vi "cic_test_reconfigure.vi"() -> ()   [LabVIEW 2013]
panel:
  out "Waveform Graph out 2":i16[](graph)
  out "Waveform Graph out":dbl[](graph)
  out "Waveform Graph":dbl[](graph)
  out "# of Iterations":i32
  out "# of samples":i32
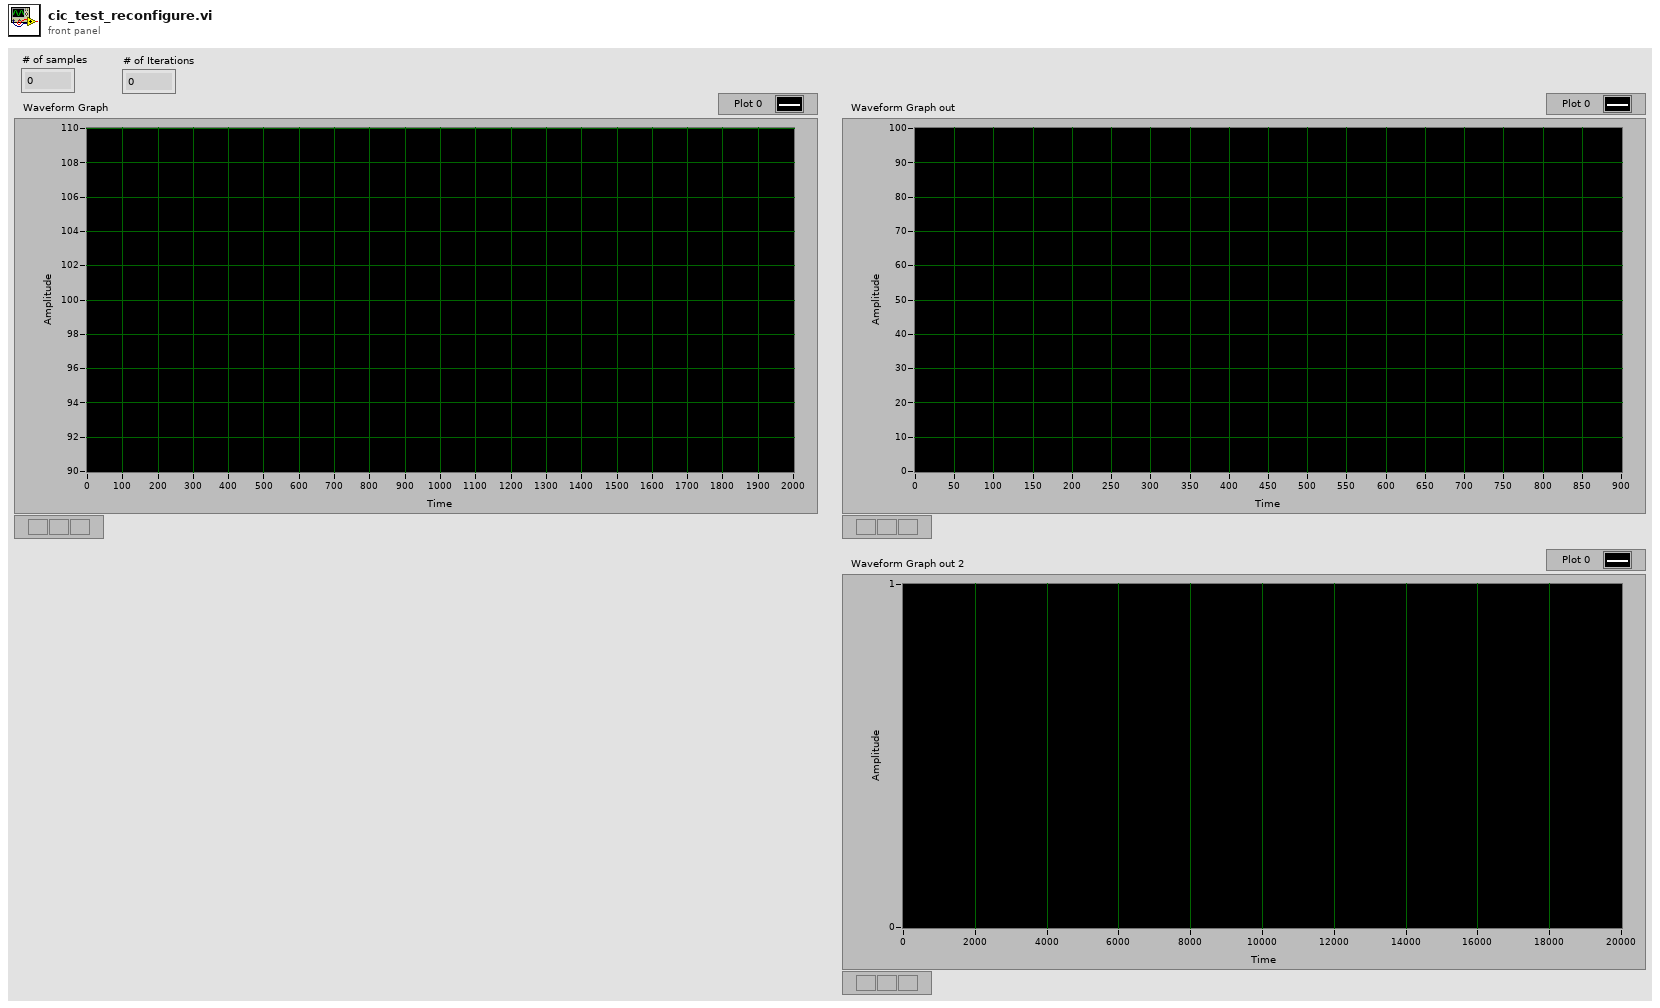
[diagram p1: front panel]
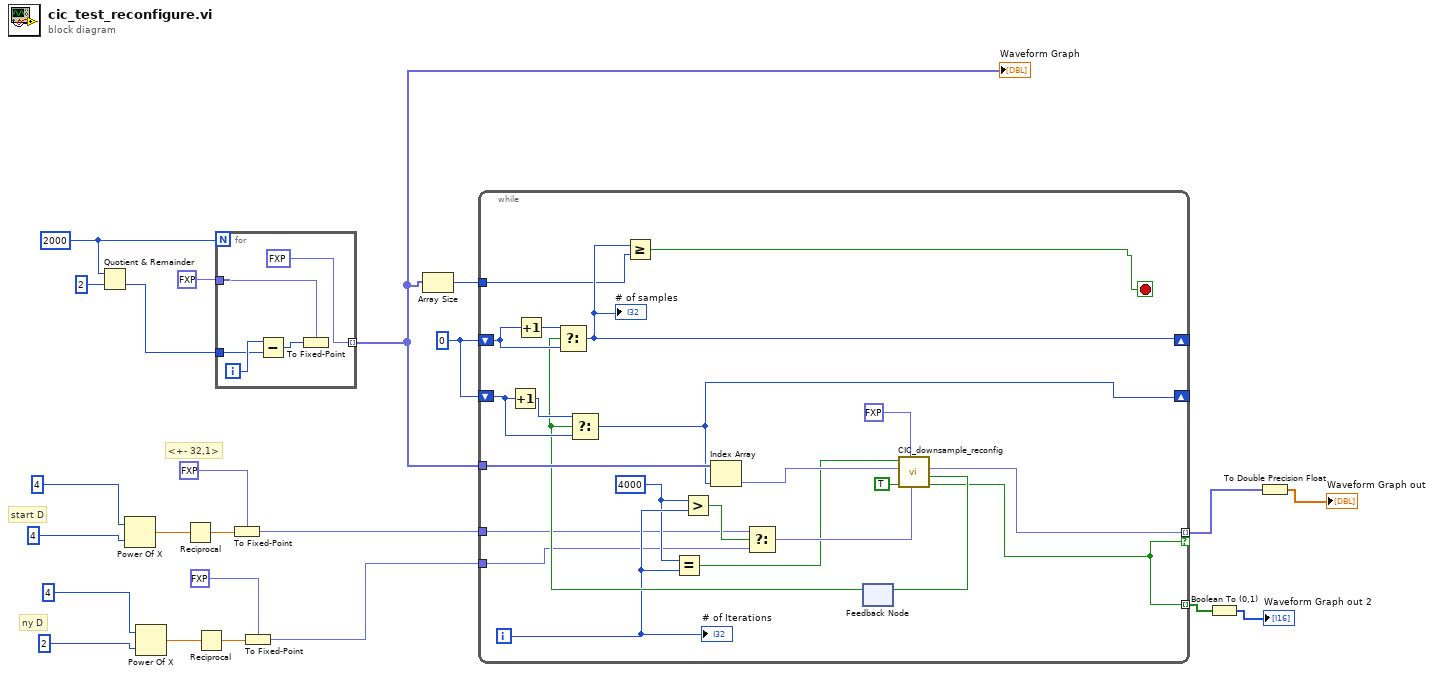
[diagram p0: block diagram]
diagram:
  w17 = 2000
  w21 = 0 ("samples")
  # "<+- 32,1>"
  # "ny D"
  # "start D"
  n1 = Quotient & Remainder(x=w17, y=2) -> (floor(x/y)=w15:i32)  [unwired: 1 out]
  n2 = Power Of X(1:4, 2:4) -> (0:w10:dbl)
  n3 = Power Of X(1:2, 2:4) -> (0:w4:dbl)
  n4 = Reciprocal(x=w10) -> (1/x=w9:dbl)
  n5 = Reciprocal(x=w4) -> (1/x=w5:dbl)
  n6 = for {
    N: w17 -> [_]
    tunnel: fxp<+/-,16,14> 0.0 ("fixed-point type") -> [w28]
    tunnel: [fxp<+/-,16,14> 100.0 ("fixed-point")] -> w18 mode=indexing
    tunnel: w15 -> [w26]
    i -> [w27]
    n7 = Subtract(x=w27, y=w26) -> (x-y=w25:i32)
    n8 = To Fixed-Point(fixed-point type=w28, number=w25) -> ()  [unwired: 1 out]
  }
  "Waveform Graph" <- w18
  n9 = To Fixed-Point(fixed-point type=fxp<+/-,32,1> 0.0 ("Gain"), number=w9) -> (fixed-point=w7:fxp<+/-,32,1>)
  n10 = To Fixed-Point(fixed-point type=fxp<+/-,32,1> 0.0 ("Gain"), number=w5) -> (fixed-point=w1:fxp<+/-,32,1>)
  n11 = Array Size(array=w18) -> (size(s)=w22:i32)
  n12 = while {
    tunnel: w18 -> [w51]
    shift-right: [w43] -> _
    shift-left: w21 -> [w49]
    shift-right: [w46] -> _
    shift-left: w21 -> [w47]
    tunnel: [w39] -> w20 mode=indexing if=w37
    tunnel: w22 -> [w44]
    tunnel: [w37] -> w14 mode=indexing
    tunnel: w7 -> [w31]
    tunnel: w1 -> [w33]
    i -> [w35]
    stop <- w45 stop-if-true
    w34 = 4000 ("x")
    n13 = Increment(x=w49) -> (x+1=w50:i32)
    n14 = Increment(x=w47) -> (x+1=w48:i32)
    n15 = Equal?(x=w34, y=w35) -> (x = y?=w29:bool)
    n16 = Greater?(x=w34, y=w35) -> (0:w32:bool)
    n17 = Select(t=w31, s=w32, f=w33) -> (s? t:f=w30:fxp<+/-,32,1>)
    n18 = feedback #1() -> (w38:bool)  [unwired: 1 in]
    n19 = Select(t=w48, s=w38, f=w47) -> (s? t:f=w46:i32)
    "# of samples" <- w46
    n20 = Select(t=w50, s=w38, f=w49) -> (s? t:f=w43:i32)
    n21 = Greater Or Equal?(x=w46, y=w44) -> (x >= y?=w45:bool)
    n22 = Index Array(array=w51, index=w43) -> (element=w42:fxp<+/-,16,14>)
    n23 = call "CIC_downsample_reconfig.vi"("Gain"=w30, "new rate"=fxp<+,8,8> 2.0, "valid in"=TRUE, "Data in"=w42, "rate change"=w29) -> ("valid out"=w37:bool, "rdy for data"=w41:bool, "dout"=w39:fxp<+/-,16,14>)  [unwired: 4 in]
    n24 = feedback-in #1(w41) -> ()
    "# of Iterations" <- w35
  }
  n25 = Boolean To (0,1)(Boolean=w14) -> (0, 1=→"Waveform Graph out 2":i16[])
  n26 = To Double Precision Float(number=w20) -> (double precision float=→"Waveform Graph out":dbl[])
